vi "Get Curr Proj Ver Index.vi"(10 "LV Proj File Path":path, 11 "LV Version Details":T1[](array[typedef])) -> (3 "Proj LV Ver Index":i32)   [LabVIEW 2016]
uses:
  controls/LV Version Details.ctl
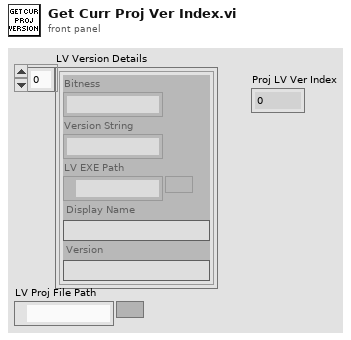
[diagram p1: front panel]
types:
  T1 = typedef "LV Version Details.ctl" = cluster{"Bitness":string, "Version String":string, "LV EXE Path":path, "Display Name":string, "Version":string}
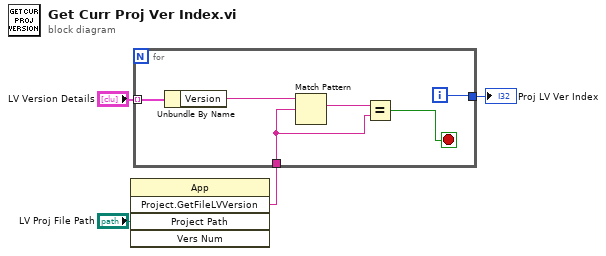
[diagram p0: block diagram]
diagram:
  n1 = invoke class="App" method="Project.GetFileLVVersion"("Project Path"="LV Proj File Path") -> ("Project.GetFileLVVersion"=w4:string)  [unwired: 4 in, 4 out]
  n2 = for {
    tunnel: "LV Version Details" -> [w10] mode=indexing
    tunnel: w4 -> [w7]
    tunnel: [w5] -> w1
    i -> [w5]
    stop <- w6 stop-if-true
    n3 = Unbundle By Name(w10) -> ("Version"=w9:string)
    n4 = Match Pattern(string=w9, regular expression=w7) -> (match substring=w8:string)  [unwired: 1 in, 3 out]
    n5 = Equal?(x=w8, y=w7) -> (x = y?=w6:bool)
  }
  "Proj LV Ver Index" <- w1
